vi "fraktal_0.vi"() -> ()   [LabVIEW 2013]
panel:
  out "2D Picture":picture
  in  "A":dbl[](array[numeric])=[0.0, 0.85, 0.2, -0.15]
  in  "F":dbl[](array[numeric])=[0.0, 1.6, 1.6, 0.44]
  in  "E":dbl[](array[numeric])=[0.0, 0.0, 0.0, 0.0]
  in  "D":dbl[](array[numeric])=[0.16, 0.85, 0.22, 0.24]
  in  "C":dbl[](array[numeric])=[0.0, -0.04, 0.23, 0.26]
  in  "B":dbl[](array[numeric])=[0.0, 0.04, -0.26, 0.28]
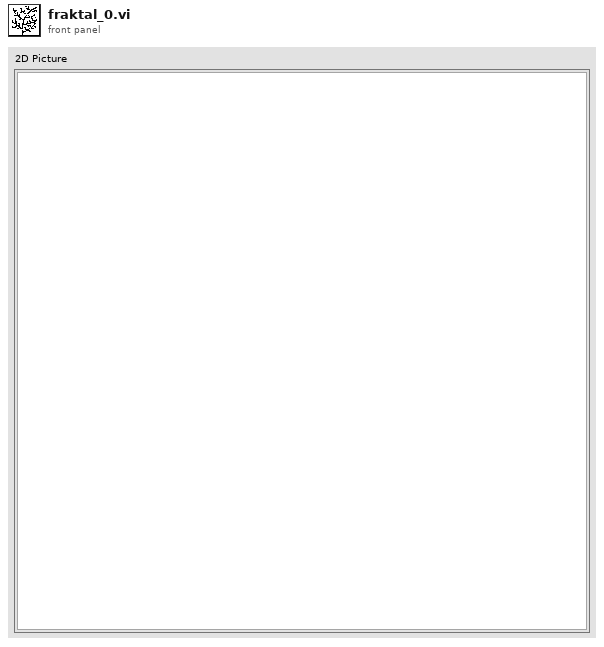
[diagram p1: front panel]
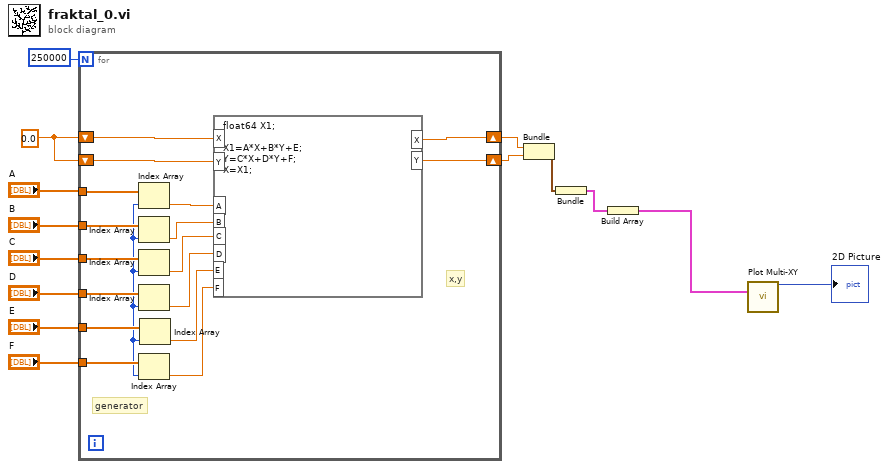
[diagram p0: block diagram]
diagram:
  w6 = 0.0
  n1 = for {
    N: 250000 -> [_]
    shift-right: [w16] -> w2
    shift-left: w6 -> [w19]
    shift-right: [w15] -> w3
    shift-left: w6 -> [w18]
    tunnel: "A" -> [w30]
    tunnel: "B" -> [w28]
    tunnel: "C" -> [w27]
    tunnel: "D" -> [w26]
    tunnel: "E" -> [w25]
    tunnel: "F" -> [w24]
    # "generator"
    # "x,y"
    n2 = Index Array(array=w28) -> (element=w29:dbl, index=w17:i32)
    n3 = Index Array(array=w30, index=w17) -> (element=w31:dbl)
    n4 = Index Array(array=w27, index=w17) -> (element=w23:dbl)
    n5 = Index Array(array=w26, index=w17) -> (element=w22:dbl)
    n6 = Index Array(array=w24, index=w17) -> (element=w20:dbl)
    n7 = Index Array(array=w25, index=w17) -> (element=w21:dbl)
    n8 = formula code="float64 X1;\n\nX1=A*X+B*Y+E;\nY=C*X+D*Y+F;\nX=X1;"("A"=w31, "X"=w19, "Y"=w18, "B"=w29, "C"=w23, "D"=w22, "E"=w21, "F"=w20) -> ("X"=w16:dbl, "Y"=w15:dbl)
  }
  n9 = Bundle(w2, w3) -> (w1:cluster{dbl, dbl})  [unwired: 1 in]
  n10 = Bundle(w1) -> (w5:cluster{cluster{dbl, dbl}})  [unwired: 1 in]
  n11 = Build Array(w5) -> (w4:cluster{cluster{dbl, dbl}}[])
  n12 = call <vilib>:"Plot Multi-XY.vi"("data"=w4) -> ("new picture"=→"2D Picture":picture)  [unwired: 14 in]
